vi "IECMemory.GetStatus.vi"(0 "i ref in":refnum<vi>, 3 "ms timeout (100)":i32=100, 5 "error in (no error)":errorcluster) -> (14 "i ref out":refnum<vi>, 16 "MemoryStatus":T1, 17 "timed out":bool, 19 "error out":errorcluster)   [LabVIEW 2014, in "IECMemory.lvlib"]
uses:
  IECMemory.lvlib
  CSCore/CSSystem/CoreDefs/CoreDefs.error_type.ctl
  CSCore/CSSystem/CoreLib/CoreLib.lvlib
  instr.lib/GPIB_Memory/Memory_Status.ctl
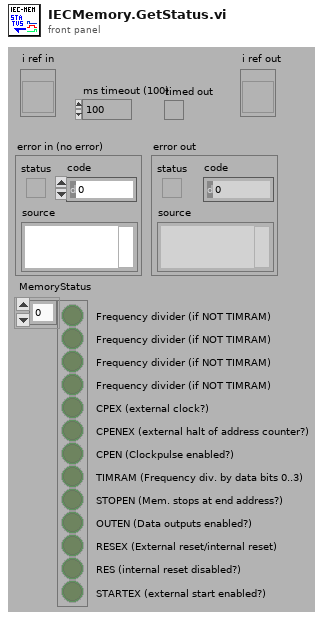
[diagram p1: front panel]
types:
  T1 = typedef "IECMemoryDriver.lvlib/Memory_Status.ctl" = bool[]
  T2 = typedef "CoreDefs.error_type.ctl" = enum16{"no error", "can't load process", "can't unload process", "process does not exist", "can't install process", "can't remove process", "unknown function", "time out", "can't execute function", "duplicate queue name", "super not found", "caller queue invalid", "can't ping process", "unknown error", "VISA Error", "VISA timeout", "GPIB timeout", "GPIB error", "communication error", "data type mismatch", "can't read data from OPC server", "can't write data to OPC server", "OET error", "function not implemented", "process already exists", "invalid Shared Variable name", "error writing Shared Variable", "error reading Shared Variable", "invalid client name", "corrupt database", "unknown class", "call not authorized", "parameter out of range", "OET timeout: can't get data to modify", "invalid queue name", "requested operation incompatible with current state", "event undefined", "event disabled", "state undefined", "caller is not a friend", "EventBuilder: bad eventID", "EventBuilder: no DAQ devices", "a thread must not stop itself", "UNUSED ELEMENT4", "DiscArchiver: eventData incomplete", "DiscArchiver: eventData does not belong to run", "DiscArchiver: can't open file", "DiscArchiver: can't write to file", "DiscArchiver: available disc space low", "can't acquire semaphore", "error reading data from database", "notifier object is not existing", "can't register process", "can't unregister process", "illegal event type", "object disabled", "object already exists", "can't change state", "Instrument not found", "no connection to remote node", "invalid reference", "N/A", "UNUSED ELEMENT 1", "element not found", "illegal TCP/IP connection detected", "object does not exist", "invalid access ID", "unknown CS system", "invalid privilige", "unsupported data type", "unsupported server type", "IO server already exists", "Shared Variable already exists"}
  T3 = typedef "IECMemory.lvlib/IECMemory.i attribute.ctl" = cluster{"EndAddress":u32, "MemoryStatusBits":T1, "IEC Finished":bool, "Call Process":string, "Call Event":string}
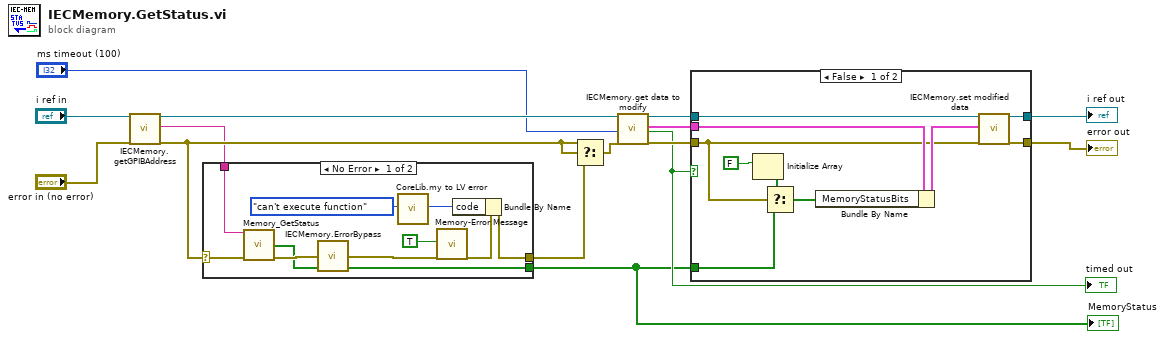
[diagram p0: block diagram]
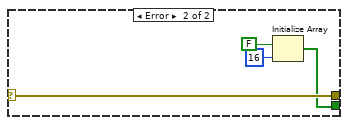
[diagram p3: hidden frame]
diagram:
  n1 = call "IECMemory.getGPIBAddress.vi"("i ref in"="i ref in", "error in (no error)"="error in (no error)") -> ("i ref out"=w12:refnum<vi>, "GPIBAddress"=w2:string, "error out"=w14:errorcluster)  [unwired: 14 in, 1 out]
  n2 = case shown="No Error" w14 {
    selector: w14 -> [w19 w29]
    tunnel: [w21 w29] -> w15
    tunnel: w2 -> [w18 _]
    tunnel: [w17 w27] -> w1
    frame No Error {
      n3 = call "Memory_GetStatus.vi"("address string"=w18, "error in"=w19) -> ("MemoryStatus"=w17:T1, "error out"=w25:errorcluster)  [unwired: 11 in, 1 out]
      n4 = call "IECMemory.ErrorBypass.vi"("error in (no error)"=w25) -> ("error out"=w16:errorcluster)  [unwired: 14 in]
      n5 = call "CoreLib.my to LV error.vi"("ErrorTypes"=CoreDefs.error_type."can't execute function") -> ("LV error code"=w20:i32)  [unwired: 17 in, 1 out]
      n6 = call "Memory-Error Message.vi"("add message to source"=TRUE, "error in (no error)"=w16) -> ("error out"=w22:errorcluster)  [unwired: 14 in, 3 out]
      n7 = Bundle By Name(cluster=w22, "code"=w20) -> (w21:errorcluster)
    }
    frame Error {
      n8 = Initialize Array(FALSE, 16 ("dimension size")) -> (w27:bool[])
    }
  }
  "MemoryStatus" <- w1
  n9 = Select(t=w14, s=w14, f=w15) -> (s? t:f=w13:errorcluster)
  n10 = call "IECMemory.get data to modify.vi"("i ref in"=w12, "ms timeout (10000)"="ms timeout (100)", "error in (no error)"=w13) -> ("i ref out"=w11:refnum<vi>, "i attribute"=w9:T3, "timed out"=w4:bool, "error out"=w10:errorcluster)  [unwired: 13 in]
  "timed out" <- w4
  n11 = case shown="False" w4 {
    tunnel: w11 -> [w33 w41]
    tunnel: [w35 w41] -> w6
    tunnel: [w34 w40] -> w5
    tunnel: w10 -> [w31 w40]
    tunnel: w9 -> [w39 _]
    tunnel: w1 -> [w30 _]
    frame False {
      n12 = Initialize Array(FALSE) -> (w37:bool[])  [unwired: 1 in]
      n13 = Select(t=w37, s=w31, f=w30) -> (s? t:f=w36:T1)
      n14 = Bundle By Name(cluster=w39, "MemoryStatusBits"=w36) -> (w32:T3)
      n15 = call "IECMemory.set modified data.vi"("i ref in"=w33, "i attribute"=w32, "error in (no error)"=w31) -> ("i ref out"=w35:refnum<vi>, "error out"=w34:errorcluster)  [unwired: 15 in]
    }
    frame True {
    }
  }
  "error out" <- w5
  "i ref out" <- w6
